vi "是否保存.vi"(1 "测试结果":string(combo)="NULL") -> (0 "保存":bool)   [LabVIEW 2020]
uses:
  <userlib>/_OpenG.lib/comparison/comparison.llb/String Changed__ogtk.vi
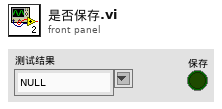
[diagram p1: front panel]
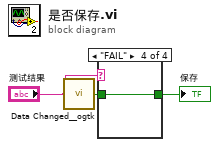
[diagram p0: block diagram]
diagram:
  n1 = call-poly <userlib>:"Data Changed__ogtk.vi"("String"="测试结果") -> ("Changed"=w1:bool)
  n2 = case shown="\"FAIL\"" "测试结果" {
    tunnel: [_ _ w4 w5] -> w3
    tunnel: w1 -> [_ _ w4 w5]
    frame "假", Default {
    }
    frame "NULL" {
    }
    frame "PASS" {
    }
    frame "FAIL" {
    }
  }
  "保存" <- w3
